vi "Demux_8.vi"(3 "Data_Array":dbl[](array[numeric]) caption="Array", 11 "Index":i32) -> (20 "element_1":dbl, 21 "element_2":dbl, 22 "element_3":dbl, 23 "element_4":dbl, 24 "element_5":dbl, 25 "element_6":dbl, 26 "element_7":dbl, 27 "element_8":dbl)   [LabVIEW 2013]
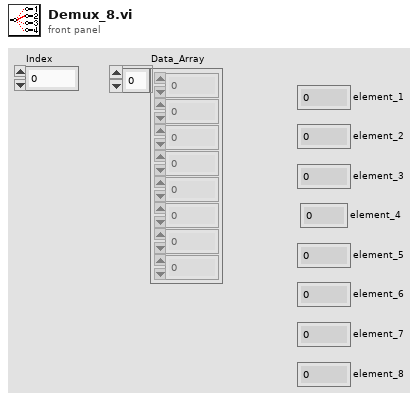
[diagram p1: front panel]
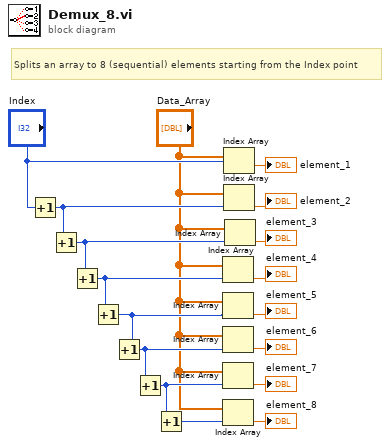
[diagram p0: block diagram]
diagram:
  # "Splits an array to 8 (sequential) elements starting from the Index point"
  n1 = Increment(x="Index") -> (x+1=w15:i32)
  n2 = Increment(x=w15) -> (x+1=w14:i32)
  n3 = Increment(x=w14) -> (x+1=w13:i32)
  n4 = Increment(x=w13) -> (x+1=w12:i32)
  n5 = Increment(x=w12) -> (x+1=w11:i32)
  n6 = Increment(x=w11) -> (x+1=w9:i32)
  n7 = Increment(x=w9) -> (x+1=w10:i32)
  n8 = Index Array(array="Data_Array", index=w13) -> (element=→"element_4":dbl)
  n9 = Index Array(array="Data_Array", index=w12) -> (element=→"element_5":dbl)
  n10 = Index Array(array="Data_Array", index=w11) -> (element=→"element_6":dbl)
  n11 = Index Array(array="Data_Array", index=w9) -> (element=→"element_7":dbl)
  n12 = Index Array(array="Data_Array", index=w10) -> (element=→"element_8":dbl)
  n13 = Index Array(array="Data_Array", index="Index") -> (element=→"element_1":dbl)
  n14 = Index Array(array="Data_Array", index=w15) -> (element=→"element_2":dbl)
  n15 = Index Array(array="Data_Array", index=w14) -> (element=→"element_3":dbl)
